vi "get channels.vi"(11 "Tagbus PID Module configuration in":refnum<class "Tagbus PID Module configuration.lvclass">) -> (2 "channels":refnum<class "TBM channel.lvclass">[](array[class]), 3 "Tagbus PID Module configuration out":refnum<class "Tagbus PID Module configuration.lvclass">)   [LabVIEW 2014, in "Tagbus PID Module configuration.lvclass"]
uses:
  Tagbus PID Module configuration.lvclass
  <vilib>/NI/Tag Bus Module Framework/channel/TBM channel.lvclass
  Tagbus PID Module configuration.lvclass/Tagbus PID Module configuration.ctl
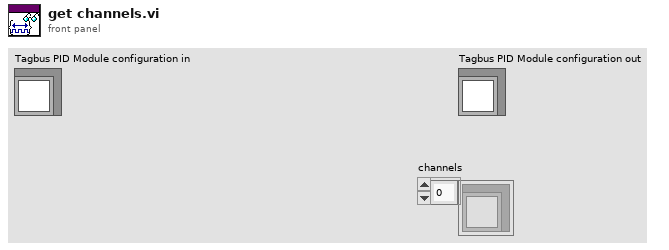
[diagram p1: front panel]
types:
  T1 = cluster{"ID":string, "Setpoint":refnum<class "TBM channel.lvclass">, "Process Variable":refnum<class "TBM channel.lvclass">, "Output":refnum<class "TBM channel.lvclass">, "PID gains":cluster{"proportional gain (Kc)":dbl, "integral time (Ti, min)":dbl, "derivative time (Td, min)":dbl}, "output range":cluster{"output high":dbl, "output low":dbl}}[]
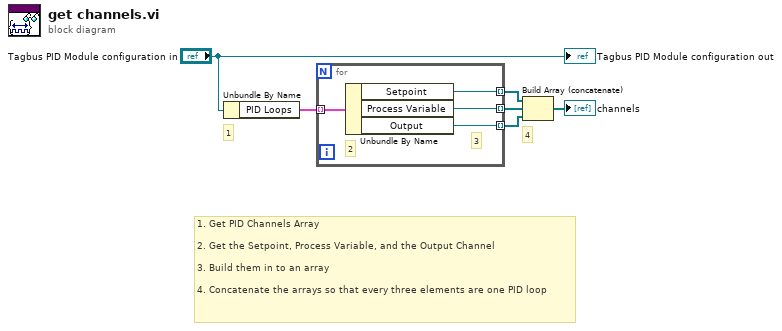
[diagram p0: block diagram]
diagram:
  # "4"
  # "1. Get PID Channels Array\n\n2. Get the Setpoint, Process Variable, and the Output Channel\n\n3. Build them in to an array\n\n4. Concatenate the arrays so that every three elements are one PID loop"
  # "1"
  n1 = Unbundle By Name("Tagbus PID Module configuration in") -> ("PID Loops"=w5:T1)
  n2 = for {
    tunnel: w5 -> [w10] mode=indexing
    tunnel: [w9] -> w3 mode=indexing
    tunnel: [w8] -> w4 mode=indexing
    tunnel: [w7] -> w2 mode=indexing
    # "3"
    # "2"
    n3 = Unbundle By Name(w10) -> ("Setpoint"=w9:refnum<class "TBM channel.lvclass">, "Process Variable"=w8:refnum<class "TBM channel.lvclass">, "Output"=w7:refnum<class "TBM channel.lvclass">)
  }
  n4 = Build Array (concatenate)(w3, w4, w2) -> (→"channels":refnum<class "TBM channel.lvclass">[])
  "Tagbus PID Module configuration out" <- "Tagbus PID Module configuration in"
